vi "Update status--all properties.vi"(4 "Background Colour":u32(colorbox)=16777215, 5 "Font size":u16, 6 "Text Colour":u32(colorbox), 7 "Font name":string, 8 "error in (no error)":errorcluster, 10 "Justification":enum16{"Left", "Center", "Right"}(ring), 11 "Text (String Value)":string) -> (0 "error out":errorcluster)   [LabVIEW 2018, in "status_text_indicator.lvlib"]
uses:
  status_text_indicator.lvlib
  PTRL/String_Control/string_control.lvlib
panel:
  # "Development\ncontrols/indicators useful for development and testing, but which are not outputs of the VI"
  # "Input\nInputs to the VI"
  # "Output\nOutputs of the VI"
  # "Description\n\nBlank VI with error handling case. \n\nSummarize the use of this VI in this space."
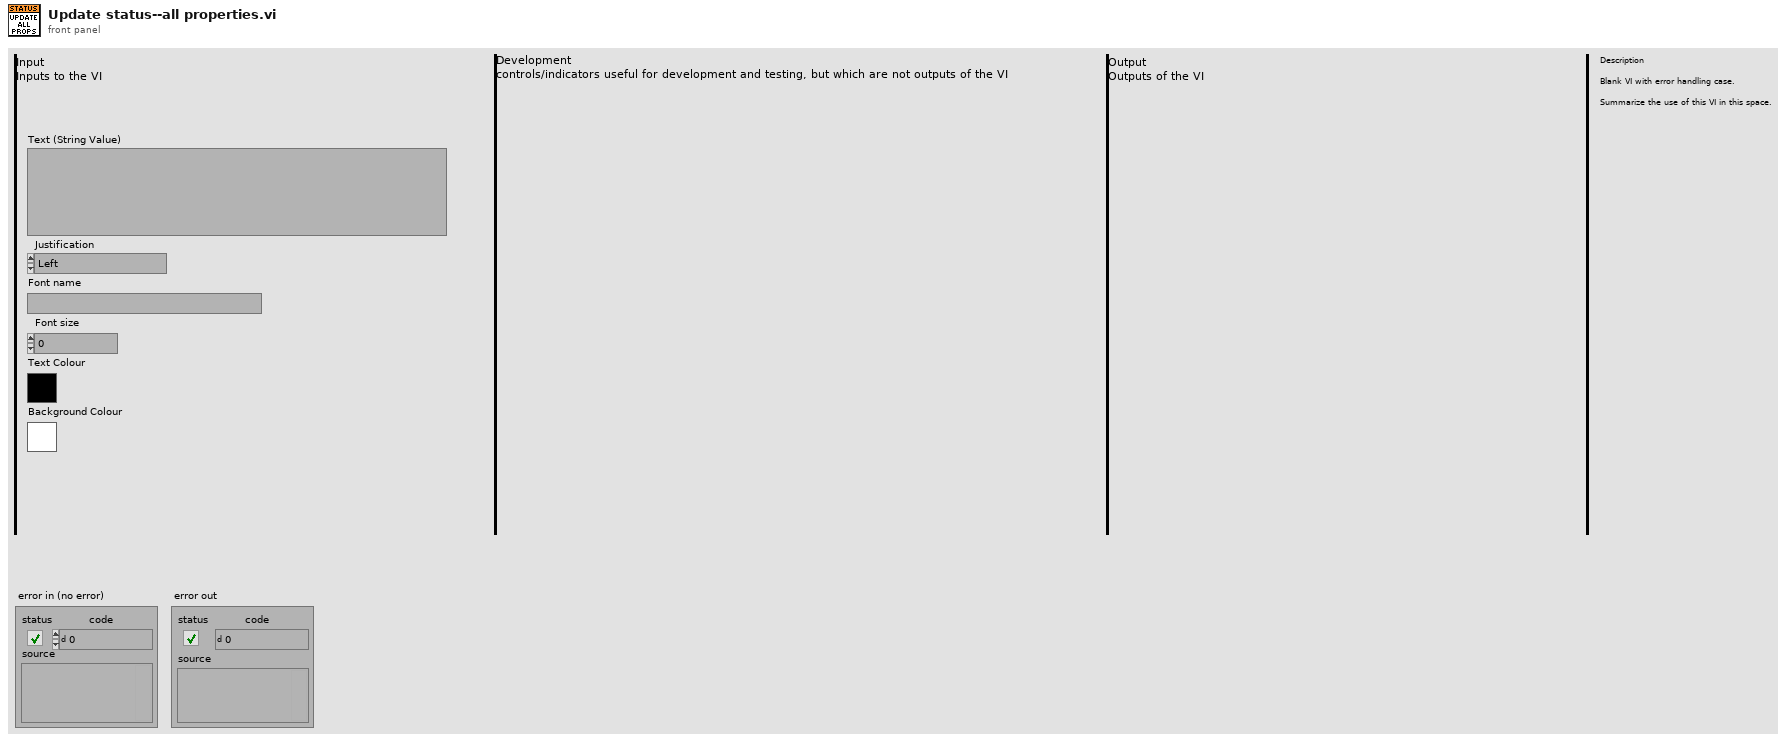
[diagram p1: front panel]
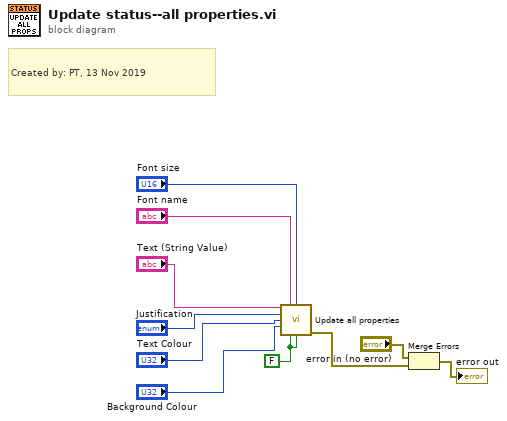
[diagram p0: block diagram]
diagram:
  w4 = FALSE ("Bold? [Default = False]")
  # "Created by: PT, 13 Nov 2019"
  n1 = call "Update all properties.vi"("String Value  [Default = \"\" (blank)]"="Text (String Value)", "Font Name [Default = \"Application Font\"]"="Font name", "Font size [Default = 15]"="Font size", "Justification [Default = Left]"="Justification", "Text Colour [Default=Pure Black=(0,0,0)]"="Text Colour", "Background Colour [Default=Pure White=(255,255,255)]"="Background Colour", "Bold? [Default = False]"=w4, "Italic? [Default = False]"=w4) -> ("error out"=w8:errorcluster)  [unwired: 7 in]
  n2 = Merge Errors("error in (no error)", w8) -> (→"error out":errorcluster)
